vi "test.vi"(1 "数值":dbl) -> (0 "数值 2":dbl)   [LabVIEW 2014]
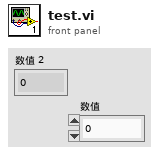
[diagram p1: front panel]
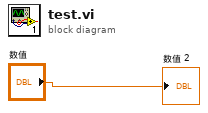
[diagram p0: block diagram]
diagram:
  "数值 2" <- "数值"
